vi "[ENO3](SubVI).vi"(8 "error in (no error)":errorcluster, 10 "ENo3-":dbl[](array[numeric]), 11 "A'":dbl[](array[numeric])) -> (0 "error out":errorcluster, 3 "[NO3]":dbl=25.057402816552635 format="%#_3g", 4 "ENo3- Graph":cluster{dbl[], dbl[]}[](graph), 5 "A'- Graph":cluster{dbl[], dbl[]}[](graph))   [LabVIEW 2019]
uses:
  Global.vi
  <vilib>/Analysis/NI_AALPro.lvlib
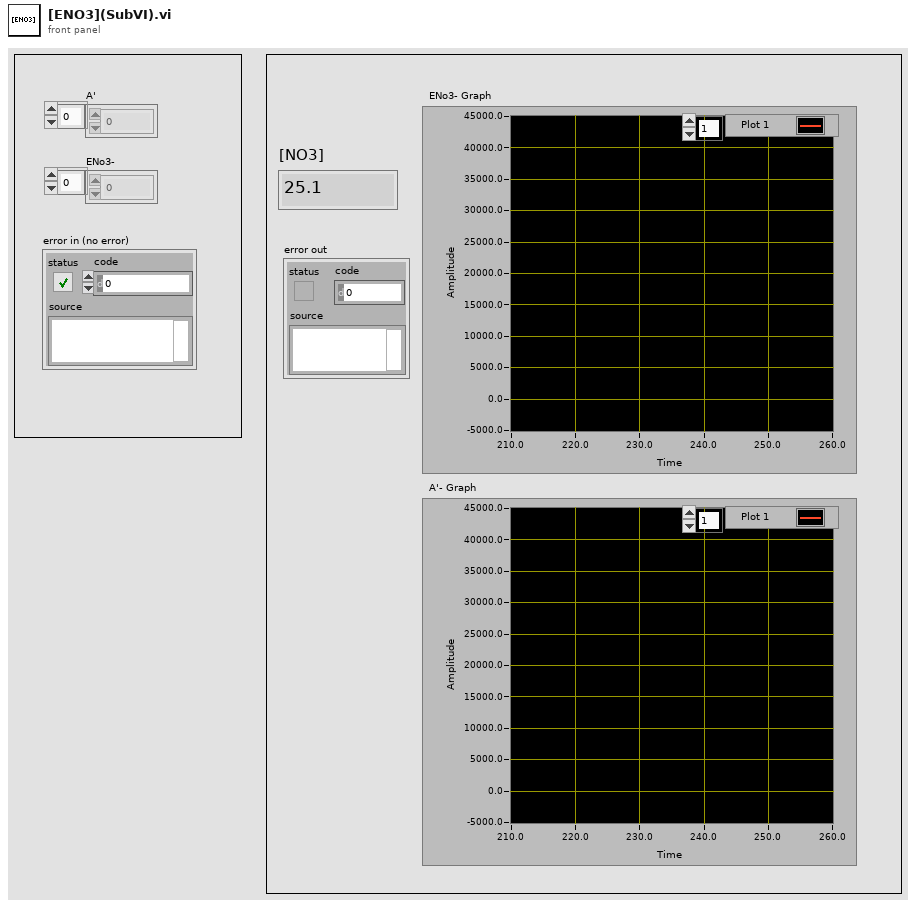
[diagram p1: front panel]
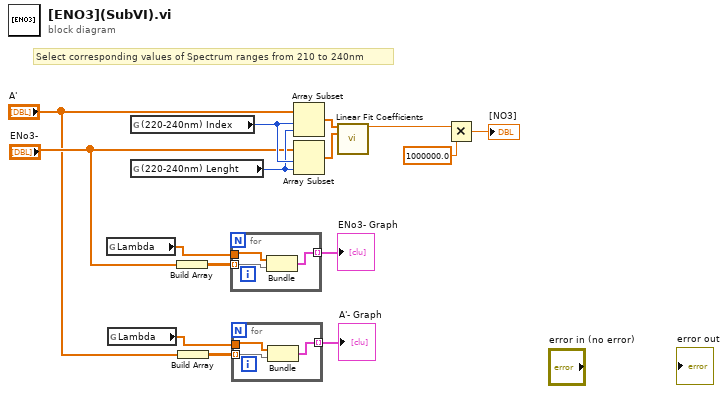
[diagram p0: block diagram]
diagram:
  # "Select corresponding values of Spectrum ranges from 210 to 240nm"
  n1 = global read "Global.vi" "Lambda"() -> (w7:dbl[])
  n2 = global read "Global.vi" "Lambda"() -> (w3:dbl[])
  n3 = global read "Global.vi" "(220-240nm) Index"() -> (w11:i32)
  n4 = global read "Global.vi" "(220-240nm) Lenght"() -> (w10:i32)
  n5 = Build Array("ENo3-") -> (w14:dbl[][])
  n6 = Build Array("A'") -> (w4:dbl[][])
  n7 = for {
    tunnel: w14 -> [w18] mode=indexing
    tunnel: [w17] -> w15 mode=indexing
    tunnel: w7 -> [w16]
    n8 = Bundle("Lambda"=w16, w18) -> (w17:cluster{"Lambda":dbl[], dbl[]})  [unwired: 1 in]
  }
  "ENo3- Graph" <- w15
  n9 = for {
    tunnel: w4 -> [w21] mode=indexing
    tunnel: [w20] -> w5 mode=indexing
    tunnel: w3 -> [w19]
    n10 = Bundle("Lambda"=w19, w21) -> (w20:cluster{"Lambda":dbl[], dbl[]})  [unwired: 1 in]
  }
  "A'- Graph" <- w5
  n11 = Array Subset(array="A'", index=w11, length=w10) -> (w8:dbl[])
  n12 = Array Subset(array="ENo3-", index=w11, length=w10) -> (w9:dbl[])
  n13 = call <vilib>:"Linear Fit Coefficients.vi"("Y"=w8, "X"=w9) -> ("slope"=w12:dbl)  [unwired: 11 in, 2 out]
  n14 = Multiply(x=w12, y=1000000.0) -> (x*y=→"[NO3]":dbl)
